vi "Start.vi"(11 "axopatch-200B in":refnum<class "axopatch-200B.lvclass">) -> (3 "axopatch-200B in 2":refnum<class "axopatch-200B.lvclass">)   [LabVIEW 2014, in "axopatch-200B.lvclass"]
uses:
  axopatch-200B.lvclass
  <vilib>/Platform/TimedLoop/XDataNode/timing_clust.ctl
  <vilib>/Platform/TimedLoop/XDataNode/nitl_modes.ctl
  <vilib>/Platform/TimedLoop/XDataNode/wakeup.ctl
  <vilib>/platform/TimedLoop/XDataNode/XDataNode.xnode
  <vilib>/Platform/TimedLoop/XDataNode/XDNodeRunTimeDep.lvlib
panel:
  out "x":dbl
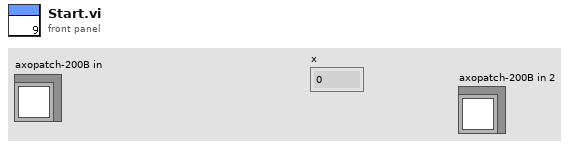
[diagram p1: front panel]
types:
  T1 = typedef "XDNodeRunTimeDep.lvlib/timing_clust.ctl" = cluster{"Expected End [f-1]":u64, "Actual End [f-1]":u64, "Finished Late? [f-1]":bool, "Expected End [i-1]":u64, "Actual End [i-1]":u64, "Finished Late? [i-1]":bool, "Expected Start [i]":u64, "Actual Start [i]":u64, "Expected Start [f]":u64, "Actual Start [f]":u64, "Source Name":string, "Structure Name":string, "Period":i64, "Deadline":i64, "Offset":i64, "Start":i64, "Priority":i32, "Timeout":i32, "Mode":T2, "Wakeup Reason":T3, "Error":errorcluster, "Source Type":string, "Secondary Source Type":string, "Global End Time":u64, "Global Start Time":u64, "Frame Duration":u64, "Iteration Duration":u64, "Assigned CPU":i32, "I/O Scan Engine Mode":u32}
  T2 = typedef "XDNodeRunTimeDep.lvlib/nitl_modes.ctl" = enum32{"No Change", "Process missed periods, maintain original phase", "Discard missed periods, maintain original phase", "Process missed periods, ignore original phase", "Discard missed periods, ignore original phase"}
  T3 = typedef "XDNodeRunTimeDep.lvlib/wakeup.ctl" = enum32{"Normal", "Aborted", "Asynchronous wakeup", "Timing source error", "Timed loop error", "Timeout"}
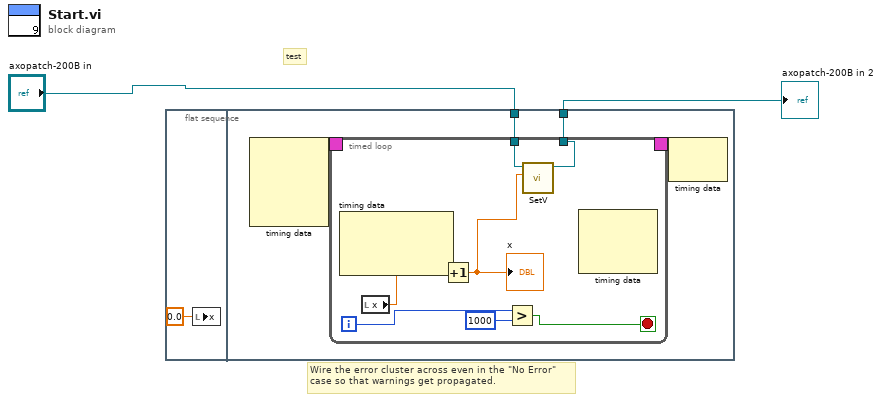
[diagram p0: block diagram]
diagram:
  # "test"
  # "Wire the error cluster across even in the \"No Error\"\ncase so that warnings get propagated."
  n1 = flat-sequence {
    tunnel: "axopatch-200B in" -> [w5]
    tunnel: [w4] -> w1
    frame #0 {
      n2 = local write "x"(0.0 ("x")) -> ()
    }
    frame #1 {
      n3 = node-c288() -> (w7:T1)  [unwired: 4 in]
      n4 = timed-loop {
        timing: w7 -> [_]
        timing-out: [_] -> w6
        tunnel: w5 -> [w10]
        tunnel: [w8] -> _
        tunnel: [w8] -> w4
        i -> [w13]
        stop <- w12 stop-if-true
        n5 = node-c288() -> ()  [unwired: 1 in, 3 out]
        n6 = local read "x"() -> (w14:dbl)
        n7 = Increment(x=w14) -> (x+1=w9:dbl)
        "x" <- w9
        n8 = Greater?(x=w13, y=1000) -> (0:w12:bool)
        n9 = call "SetV.vi"("test"=w9, "axopatch-200B in"=w10) -> ("axopatch-200B out"=w8:refnum<class "axopatch-200B.lvclass">)  [unwired: 8 in, 1 out]
        n10 = node-c288() -> ()  [unwired: 3 in, 1 out]
      }
      n11 = node-c288(w6) -> ()  [unwired: 1 out]
    }
  }
  "axopatch-200B in 2" <- w1
